vi "test_timer2.vi"() -> ()   [LabVIEW 2019]
panel:
  out "cnt":i32
  out "time_status_out":T1 {"total time" format="%.1f"; "run time" format="%.1f"; "pause time" format="%.1f"}
  out "time-out":bool
  in  "stop":bool
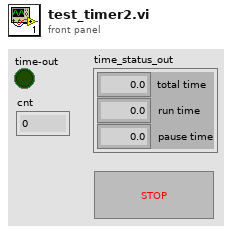
[diagram p1: front panel]
types:
  T1 = cluster{"total time":dbl, "run time":dbl, "pause time":dbl}
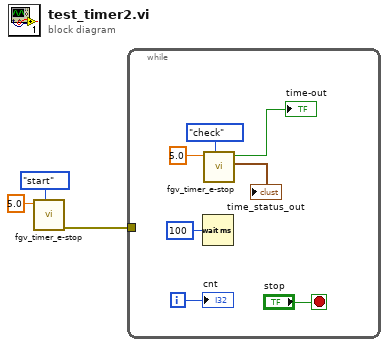
[diagram p0: block diagram]
diagram:
  n1 = call "fgv_timer_e-stop.vi"("cmd"=enum16{"check", "start", "pause"}."start", "target time"=5.0) -> ("error out"=w1:errorcluster)  [unwired: 7 in, 2 out]
  n2 = while {
    tunnel: w1 -> [_]
    i -> [w4]
    stop <- "stop" stop-if-true
    n3 = Wait (ms)(milliseconds to wait=u32 100) -> ()  [unwired: 1 out]
    n4 = call "fgv_timer_e-stop.vi"("cmd"=enum16{"check", "start", "pause"}."check", "target time"=5.0) -> ("time_status_out"=→"time_status_out":T1, "time-out"=→"time-out":bool)  [unwired: 7 in, 1 out]
    "cnt" <- w4
  }
